vi "Light Sensor.vi"() -> ()   [LabVIEW 2014]
uses:
  <vilib>/_DAQmxBase/Internals/DAQmxBase Read (Analog 1D DBL NChan 1Samp).vi
panel:
  out "C":dbl
  out "B":dbl
  out "A":dbl
  out "Distance":dbl
  out "Sum":dbl
  out "Average":dbl
  out "Current Value":dbl
  in  "loops":i32
  out "error out":errorcluster
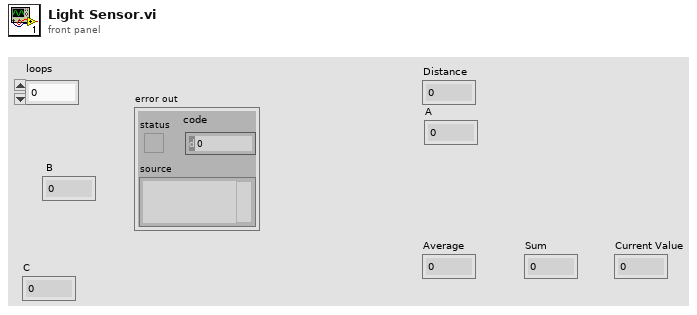
[diagram p1: front panel]
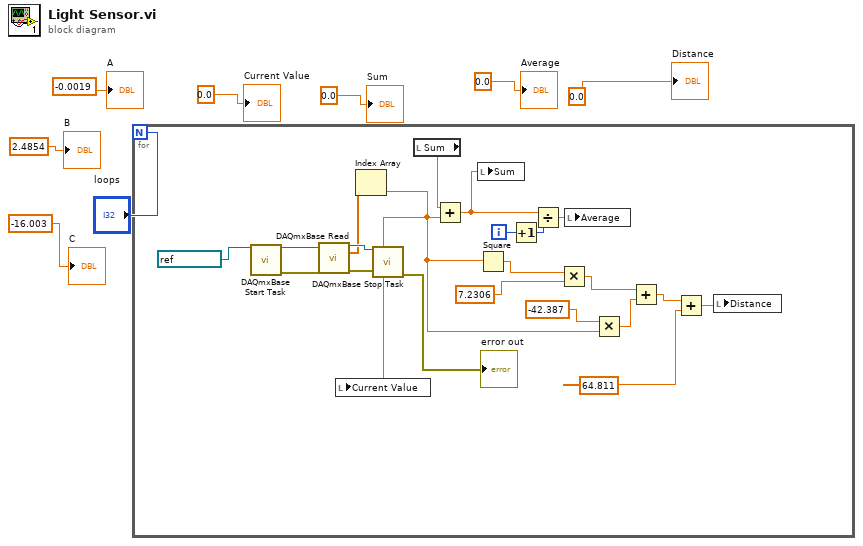
[diagram p0: block diagram]
diagram:
  n1 = for {
    N: "loops" -> [_]
    i -> [w21]
    n2 = call <vilib>:"DAQmxBase Start Task.vi"("task/channels in"=refnum<k21> "voltage" ("DAQmx Task Name")) -> ("task out"=w26:refnum<k21>, "error out"=w28:errorcluster)  [unwired: 13 in]
    n3 = call-poly <vilib>:"DAQmxBase Read.vi"("task/channels in"=w26, "error in"=w28) -> ("task out"=w24:refnum<k21>, "data"=w23:dbl[], "error out"=w27:errorcluster)  [unwired: 11 in]
    n4 = Index Array(array=w23) -> (element=w14:dbl)  [unwired: 1 in]
    n5 = local write "Current Value"(w14) -> ()
    n6 = call <vilib>:"DAQmxBase Stop Task.vi"("task/channels in"=w24, "error in"=w27) -> ("error out"=→"error out":errorcluster)  [unwired: 12 in, 1 out]
    n7 = local read "Sum"() -> (w22:dbl)
    n8 = Add(x=w22, y=w14) -> (x+y=w18:dbl)
    n9 = local write "Sum"(w18) -> ()
    n10 = Square(x=w14) -> (x^2=w17:dbl)
    n11 = Increment(x=w21) -> (x+1=w20:i32)
    n12 = Divide(x=w18, y=w20) -> (x/y=w19:dbl)
    n13 = Multiply(x=w17, y=7.2306) -> (x*y=w16:dbl)
    n14 = local write "Average"(w19) -> ()
    n15 = Multiply(x=-42.387, y=w14) -> (x*y=w15:dbl)
    n16 = Add(x=w16, y=w15) -> (x+y=w13:dbl)
    n17 = Add(x=w13, y=64.811) -> (x+y=w9:dbl)
    n18 = local write "Distance"(w9) -> ()
  }
  "Current Value" <- 0.0
  "Average" <- 0.0
  "Sum" <- 0.0
  "Distance" <- 0.0
  "A" <- -0.0019
  "B" <- 2.4854
  "C" <- -16.003
